vi "Add Path.vi"(7 "Grid Size (10)":i32=10, 8 "Path In":picture, 9 "Old Position":T1, 10 "New Position":T1) -> (0 "Path":picture)   [LabVIEW 2020, in "App.lvlib" / "MazeUI.lvclass"]
uses:
  MazeUI.lvclass
  Maze/Position.ctl
  Maze/Maze.lvlib
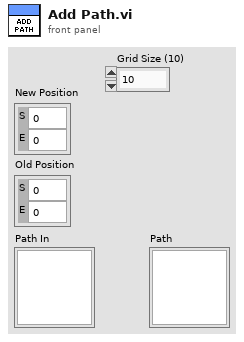
[diagram p1: front panel]
types:
  T1 = typedef "Maze.lvlib/Position.ctl" = cluster{"S":i32, "E":i32}
  T2 = cluster{"Width":u16, "Style":enum32{"Solid", "Dash", "Dot", "DashDot", "DashDotDot"}}
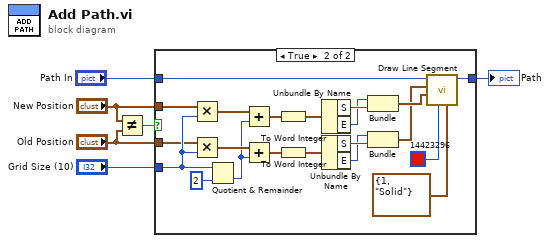
[diagram p0: block diagram]
diagram:
  n1 = Not Equal?(x="New Position", y="Old Position") -> (x != y?=w1:bool)
  n2 = case shown="True" w1 {
    tunnel: "Path In" -> [w7 w27]
    tunnel: [w7 w26] -> w5
    tunnel: "Grid Size (10)" -> [_ w24]
    tunnel: "New Position" -> [_ w9]
    tunnel: "Old Position" -> [_ w8]
    frame False {
    }
    frame True {
      n3 = Multiply(x=w9, y=w24) -> (x*y=w23:T1)
      n4 = Multiply(x=w8, y=w24) -> (x*y=w22:T1)
      n5 = Quotient & Remainder(x=w24, y=2) -> (floor(x/y)=w21:i32)  [unwired: 1 out]
      n6 = Add(x=w23, y=w21) -> (x+y=w20:T1)
      n7 = Add(x=w22, y=w21) -> (x+y=w19:T1)
      n8 = To Word Integer(number=w20) -> (16bit integer=w18:cluster{"S":i16, "E":i16})
      n9 = To Word Integer(number=w19) -> (16bit integer=w17:cluster{"S":i16, "E":i16})
      n10 = Unbundle By Name(w18) -> ("S"=w16:i16, "E"=w15:i16)
      n11 = Unbundle By Name(w17) -> ("S"=w13:i16, "E"=w12:i16)
      n12 = Bundle("E"=w15, "S"=w16) -> (w14:cluster{"E":i16, "S":i16})  [unwired: 1 in]
      n13 = Bundle("E"=w12, "S"=w13) -> (w11:cluster{"E":i16, "S":i16})  [unwired: 1 in]
      n14 = call "Draw Line Segment.vi"("pen"=T2 {"Width"=1, "Style"=enum."Solid"}, "color"=u32 14423296, "End"=w14, "Start"=w11, "Picture In (New)"=w27) -> ("Picture"=w26:picture)  [unwired: 6 in]
    }
  }
  "Path" <- w5
